vi "Initialize.vi"(8 "error in":errorcluster, 10 "shared resources":refnum<class "Shared Resources.lvclass">, 11 "logging execution unit in":refnum<class "Logging Execution Unit.lvclass">) -> (0 "error out":errorcluster, 3 "logging execution unit out":refnum<class "Logging Execution Unit.lvclass">)   [LabVIEW 2023, in "Ballard MIL-STD-1553 Engine Support.lvlib" / "Implementation.lvlib" / "Logging Execution Unit.lvclass"]
uses:
  Logging Execution Unit.lvclass
  C:/dev/CD/niveristand-ballard-milStd1553-custom-device/Source/Custom Device Support/Engine/Implementation/Execution Unit/Execution Unit.lvclass
  Interfaces/Shared Resources/Shared Resources.lvclass
  Shared Resources/Shared Resources.lvclass
  Logging Execution Unit.lvclass/Logging Execution Unit.ctl
  Execution Unit/Execution Unit.lvclass/Execution Unit.ctl
  Execution Unit/Execution Unit.lvclass
  <instrlib>/BTICardLib/BTICardLV.lvlib
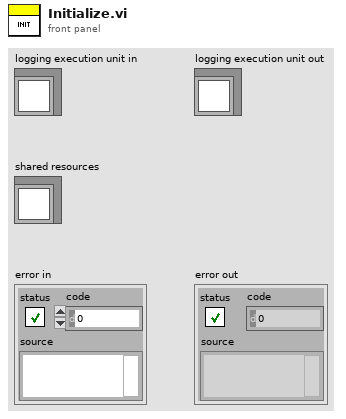
[diagram p1: front panel]
types:
  T1 = typedef "Ballard MIL-STD-1553 Engine Support.lvlib/Custom Device.lvlib/Hardware Handles.ctl" = cluster{"core handle":u64, "core reader handle":u64, "channel handles":u64[]}
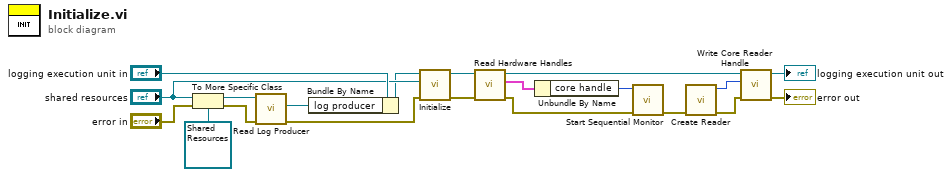
[diagram p0: block diagram]
diagram:
  n1 = To More Specific Class(target class=refnum<class "Shared Resources.lvclass"> refnum ("Shared Resources in"), reference="shared resources", error in="error in") -> (specific class reference=w12:refnum<class "Shared Resources.lvclass">, error out=w18:errorcluster)
  n2 = call-dynamic "Read Log Producer.vi"("error in (no error)"=w18, "Shared Resources in"=w12) -> ("error out"=w20:errorcluster, "Communication Bus Template Interfaces:Implementation.lvlib:Word Logging.lvlib:Log Producer.lvclass"=w16:refnum<class "Log Producer.lvclass">)  [unwired: 7 in, 1 out]
  n3 = Bundle By Name(cluster="logging execution unit in", "log producer"=w16) -> (w1:refnum<class "Logging Execution Unit.lvclass">)
  n4 = call-parent "Initialize.vi"("error in"=w20, "shared resources"="shared resources", "Execution Unit Implementation in"=w1) -> ("error out"=w10:errorcluster, "Execution Unit Implementation out"=w11:refnum<class "Logging Execution Unit.lvclass">)  [unwired: 7 in]
  n5 = call "Read Hardware Handles.vi"("error in"=w10, "Execution Unit in"=w11) -> ("error out"=w7:errorcluster, "hardware handles"=w9:T1, "Execution Unit out"=w2:refnum<class "Logging Execution Unit.lvclass">)  [unwired: 7 in]
  n6 = Unbundle By Name(w9) -> ("core handle"=w8:u64)
  n7 = call <instrlib>:"Start Sequential Monitor.vi"("error in (no error)"=w7, "core handle in"=w8) -> ("error out"=w14:errorcluster)  [unwired: 8 in, 1 out]
  n8 = call <instrlib>:"Create Reader.vi"("error in (no error)"=w14) -> ("error out"=w5:errorcluster, "core reader handle out"=w3:u64)  [unwired: 9 in]
  n9 = call "Write Core Reader Handle.vi"("error in"=w5, "core reader handle"=w3, "execution unit in"=w2) -> ("error out"=→"error out":errorcluster, "execution unit out"=→"logging execution unit out":refnum<class "Logging Execution Unit.lvclass">)  [unwired: 7 in]
